vi "PipelineDuty1.vi"(8 "error in (no error)":errorcluster, 10 "DataExchange":T1, 11 "GRMActor in":refnum<class "DisplayerUI.lvclass">) -> (0 "error out":errorcluster, 2 "DataExchange Out":T1, 3 "GRMActor out":refnum<class "DisplayerUI.lvclass">)   [LabVIEW 2020]
uses:
  DisplayerUI.lvclass
  Hardware Abstraction Layer/Component/Device/Device/DataExchange.ctl
  Interface/DataListener/DataListener.lvclass
panel:
  out "Source":string
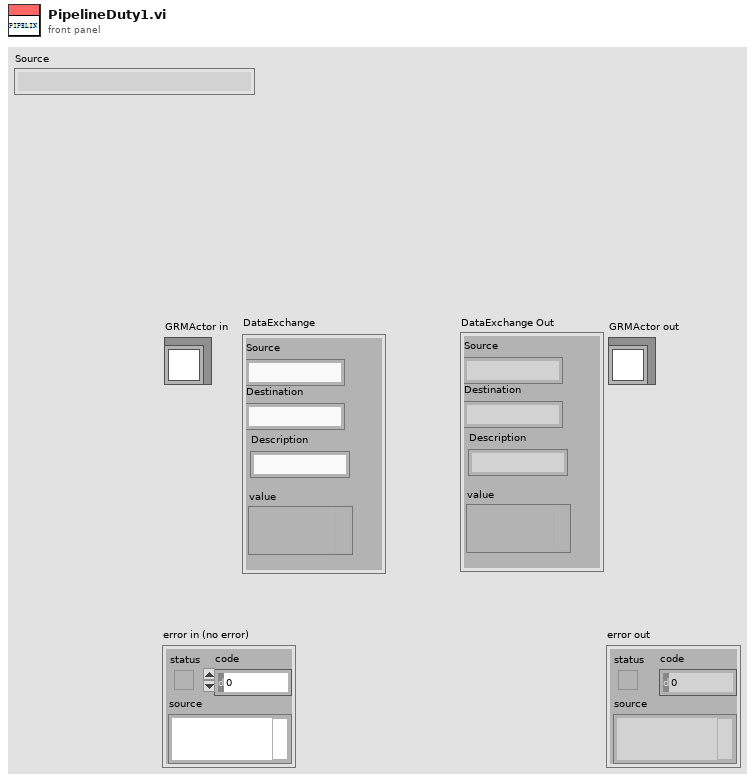
[diagram p1: front panel]
types:
  T1 = typedef "DataListener.lvclass/DataExchange.ctl" = cluster{"Source":string, "Destination":string, "Description":string, "value":variant}
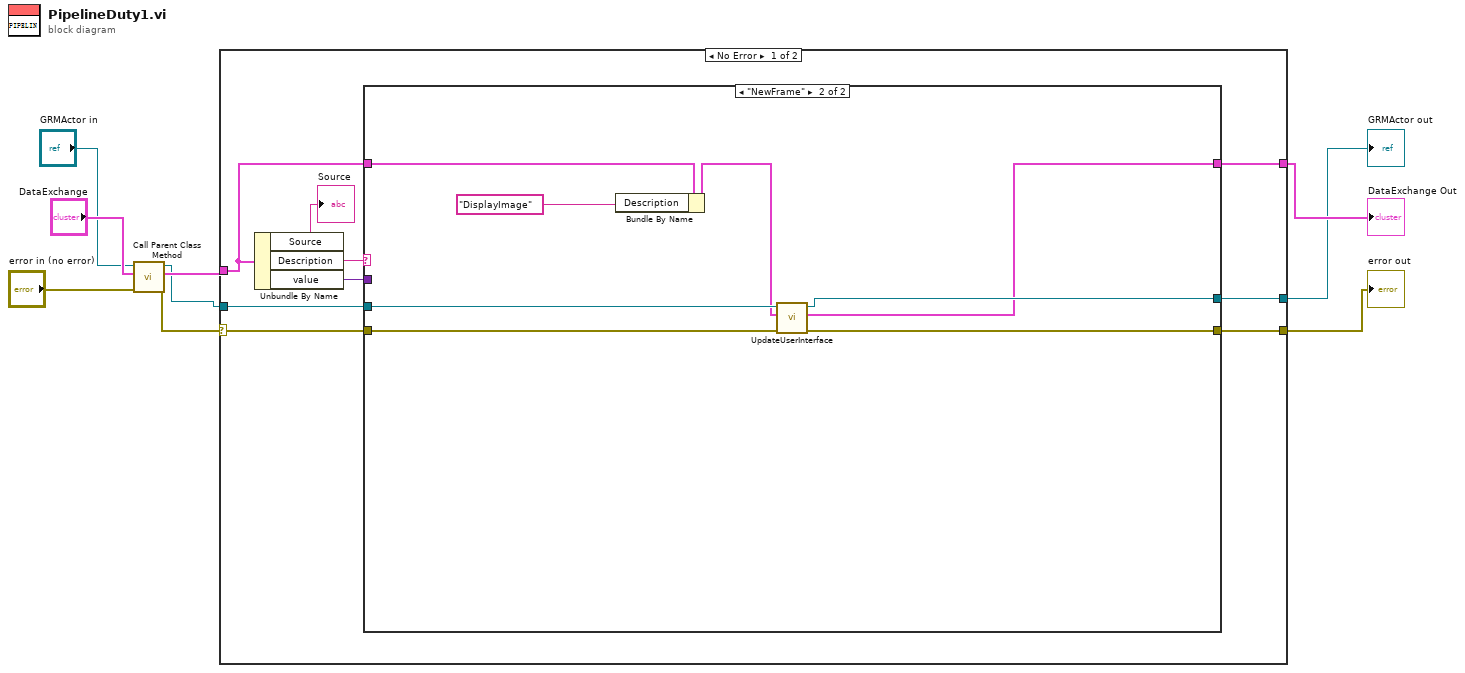
[diagram p0: block diagram]
diagram:
  n1 = call-parent "Call Parent Class Method"("error in (no error)"="error in (no error)", "DataExchange"="DataExchange", "GRMActor in"="GRMActor in") -> ("error out"=w4:errorcluster, "DataExchange Out"=w6:T1, "GRMActor out"=w5:refnum<class "DisplayerUI.lvclass">)  [unwired: 6 in]
  n2 = case shown="No Error" w4 {
    selector: w4 -> [w16 w32]
    tunnel: [w17 w32] -> w1
    tunnel: w5 -> [w13 w31]
    tunnel: [w18 w31] -> w2
    tunnel: w6 -> [w12 w30]
    tunnel: [w11 w30] -> w3
    frame No Error {
      n3 = Unbundle By Name(w12) -> ("Source"=→"Source":string, "Description"=w15:string, "value"=w14:variant)
      n4 = case shown="\"NewFrame\"" w15 {
        tunnel: w14 -> [_ _]
        tunnel: [w21 w26] -> w18
        tunnel: w13 -> [w21 w27]
        tunnel: [w20 w28] -> w17
        tunnel: w16 -> [w20 w29]
        tunnel: w12 -> [w19 w25]
        tunnel: [w19 w24] -> w11
        frame Default {
        }
        frame "NewFrame" {
          n5 = Bundle By Name(cluster=w25, "Description"="DisplayImage") -> (w23:T1)
          n6 = call-dynamic "UpdateUserInterface.vi"("error in (no error)"=w29, "DataExchange"=w23, "DisplayerUI in"=w27) -> ("error out"=w28:errorcluster, "DataExchange Out"=w24:T1, "DisplayerUI out"=w26:refnum<class "DisplayerUI.lvclass">)  [unwired: 6 in]
        }
      }
    }
    frame Error {
    }
  }
  "error out" <- w1
  "GRMActor out" <- w2
  "DataExchange Out" <- w3
